vi "Setting FP Controls.vi"(3 "error out":errorcluster, 4 "This VI":refnum<vi>, 5 "Control Value:Get All":cluster{"Name":string, "Variant Data":variant}[](array[cluster])) -> (0 "error out 2":errorcluster)   [LabVIEW 2013]
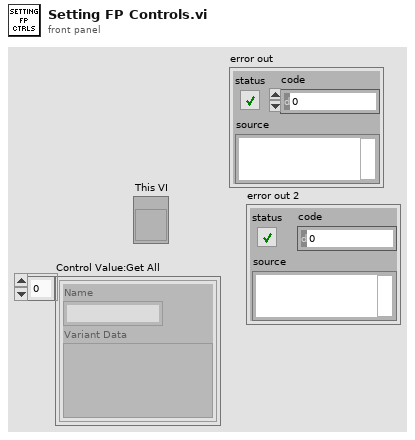
[diagram p1: front panel]
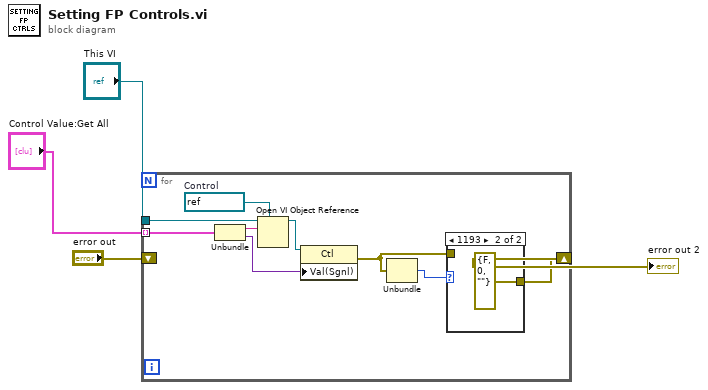
[diagram p0: block diagram]
diagram:
  n1 = for {
    shift-right: [w6] -> w3
    shift-left: "error out" -> [_]
    tunnel: "This VI" -> [w11]
    tunnel: "Control Value:Get All" -> [w13] mode=indexing
    w8 = refnum<vi> refnum  # Control
    n2 = Unbundle(w13) -> ("Name"=w10:string, "Variant Data"=w12:variant)
    n3 = Open VI Object Reference(7:w8, 10:w10, 11:w11) -> (3:w9:refnum<vi>)  [unwired: 1 in, 1 out]
    n4 = property class="Ctl"(reference=w9, "Val(Sgnl)"=w12) -> (error out=w5:errorcluster)  [unwired: 1 in, 1 out]
    n5 = Unbundle(w5) -> ("code"=w7:i32)  [unwired: 2 out]
    n6 = case shown="1193" w7 {
      tunnel: [w14 errorcluster {"status"=FALSE, "code"=0, "source"=""} ("error constant")] -> w6
      tunnel: w5 -> [w14 _]
      frame 0, Default {
      }
      frame 1193 {
      }
    }
  }
  "error out 2" <- w3
